vi "get.all.tests.directories.vi"(8 "error in":errorcluster, 10 "filter":string="tests", 11 "Path.in":path) -> (0 "error out":errorcluster, 3 "Test Directories":path[](array[path]))   [LabVIEW 2022 SP3]
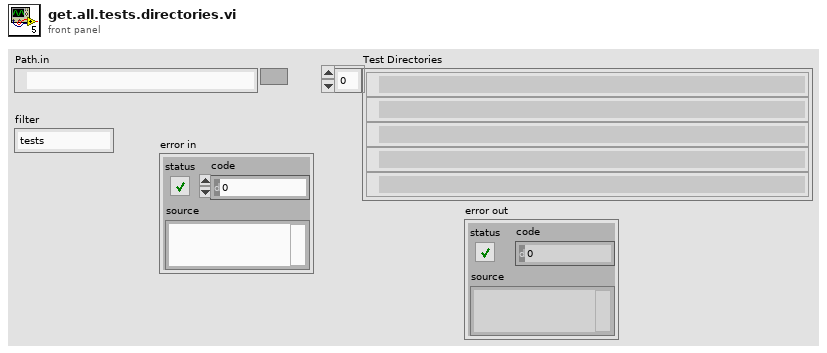
[diagram p1: front panel]
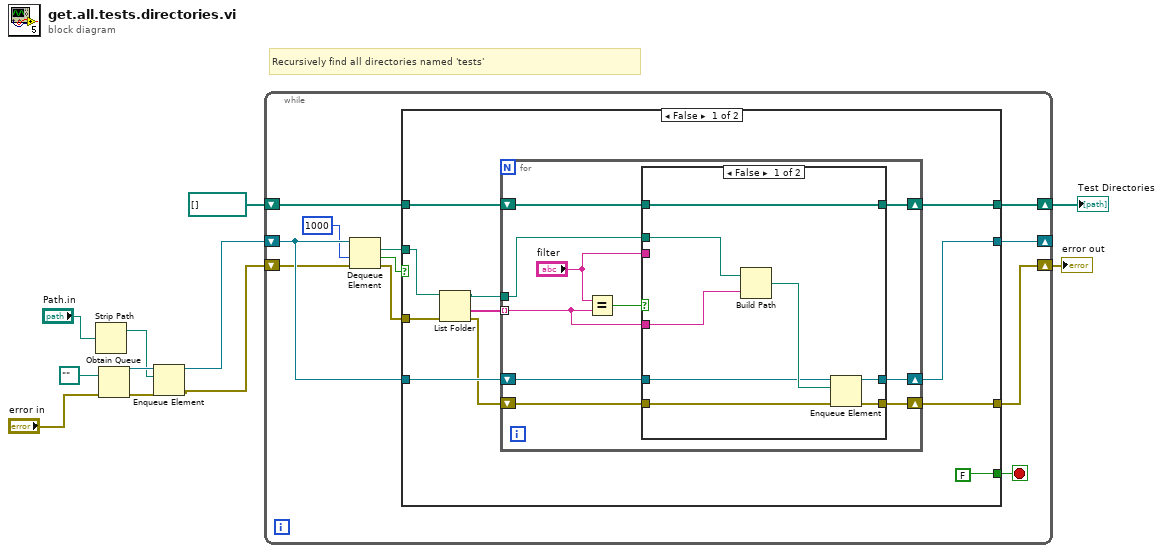
[diagram p0: block diagram]
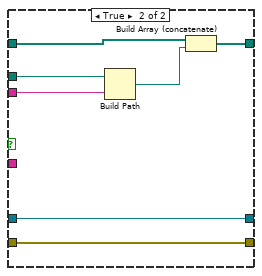
[diagram p2: hidden frame]
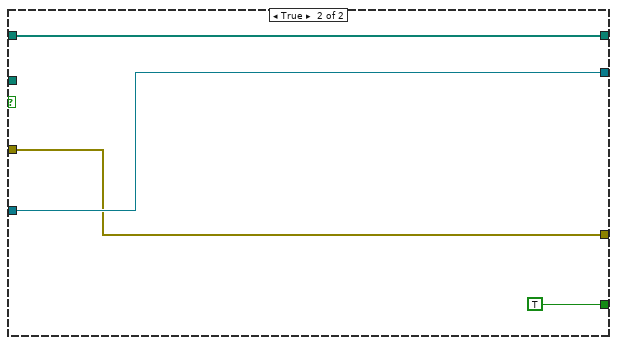
[diagram p3: hidden frame]
diagram:
  # "Recursively find all directories named 'tests'"
  n1 = Strip Path(path="Path.in") -> (stripped path=w8:path)  [unwired: 1 out]
  n2 = Obtain Queue(element data type=path "" ("stripped path"), error in (no error)="error in") -> (queue out=w9:refnum<queue>, error out=w3:errorcluster)  [unwired: 3 in, 1 out]
  n3 = Enqueue Element(queue=w9, element=w8, error in (no error)=w3) -> (queue out=w6:refnum<queue>, error out=w2:errorcluster)  [unwired: 1 in, 1 out]
  n4 = while {
    shift-right: [w22] -> w11
    shift-left: path[] [] -> [w20]
    shift-right: [w17] -> _
    shift-left: w6 -> [w16]
    shift-right: [w12] -> w1
    shift-left: w2 -> [w14]
    stop <- w18 stop-if-true
    n5 = Dequeue Element(queue=w16, timeout in ms (-1)=1000, error in (no error)=w14) -> (element=w21:path, timed out?=w19:bool, error out=w13:errorcluster)  [unwired: 1 out]
    n6 = case shown="False" w19 {
      tunnel: [w32 w61] -> w22
      tunnel: w21 -> [w30 _]
      tunnel: w20 -> [w29 w61]
      tunnel: [FALSE TRUE] -> w18
      tunnel: [w26 w60] -> w17
      tunnel: w16 -> [w27 w60]
      tunnel: w13 -> [w25 w59]
      tunnel: [w23 w59] -> w12
      frame False {
        n7 = List Folder(path=w30, error in=w25) -> (path out=w31:path, folder names=w33:string[], error out=w24:errorcluster)  [unwired: 2 in, 1 out]
        n8 = for {
          tunnel: w33 -> [w36] mode=indexing
          shift-right: [w41] -> w32
          shift-left: w29 -> [w42]
          tunnel: w31 -> [w40]
          shift-right: [w37] -> w26
          shift-left: w27 -> [w38]
          shift-right: [w34] -> w23
          shift-left: w24 -> [w35]
          n9 = Equal?(x="filter", y=w36) -> (x = y?=w43:bool)
          n10 = case shown="False" w43 {
            tunnel: w42 -> [w51 w58]
            tunnel: [w51 w57] -> w41
            tunnel: w40 -> [w50 w56]
            tunnel: "filter" -> [_ w55]
            tunnel: w38 -> [w48 w53]
            tunnel: [w47 w53] -> w37
            tunnel: w36 -> [w46 _]
            tunnel: w35 -> [w45 w52]
            tunnel: [w44 w52] -> w34
            frame False {
              n11 = Build Path(base path=w50, name or relative path=w46) -> (appended path=w49:path)
              n12 = Enqueue Element(queue=w48, element=w49, error in (no error)=w45) -> (queue out=w47:refnum<queue>, error out=w44:errorcluster)  [unwired: 1 in, 1 out]
            }
            frame True {
              n13 = Build Path(base path=w56, name or relative path=w55) -> (appended path=w54:path)
              n14 = Build Array (concatenate)(w58, w54) -> (w57:path[])
            }
          }
        }
      }
      frame True {
      }
    }
  }
  "Test Directories" <- w11
  "error out" <- w1
